vi "Draw Flat Top Textured Triangle.vi"(0 "Texture 3":T2, 4 "Texture 2":T2, 6 "Texture 1":T2, 8 "Point 3":T2, 9 "Point 2":T2, 10 "Point 1":T2, 11 "Pixel Data in":u32[][](array[numeric])) -> (3 "Pixel Data out":u32[][](array[numeric]))   [LabVIEW 2022 SP3]
uses:
  Point 2D.ctl
  Raster.lvlib
  Method.ctl
  <vilib>/picture/picture.llb/imagedata.ctl
panel:
  in  "Texture":T1
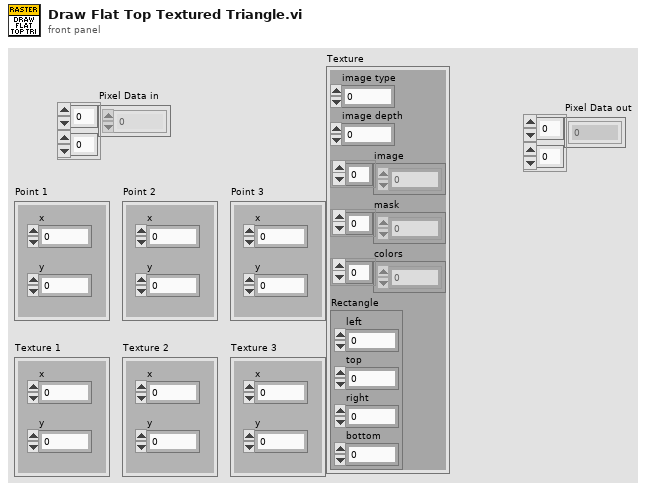
[diagram p1: front panel]
types:
  T1 = typedef "imagedata.ctl" = cluster{"image type":i32, "image depth":i32, "image":u8[], "mask":u8[], "colors":u32[], "Rectangle":cluster{"left":i16, "top":i16, "right":i16, "bottom":i16}}
  T2 = typedef "Raster.lvlib/Point 2D.ctl" = cluster{"x":i32, "y":i32}
  T3 = typedef "Raster.lvlib/Method.ctl" = enum16{"Per item", "Row", "Replace Array Subset", "MoveBlock", " MoveBlock2 "}
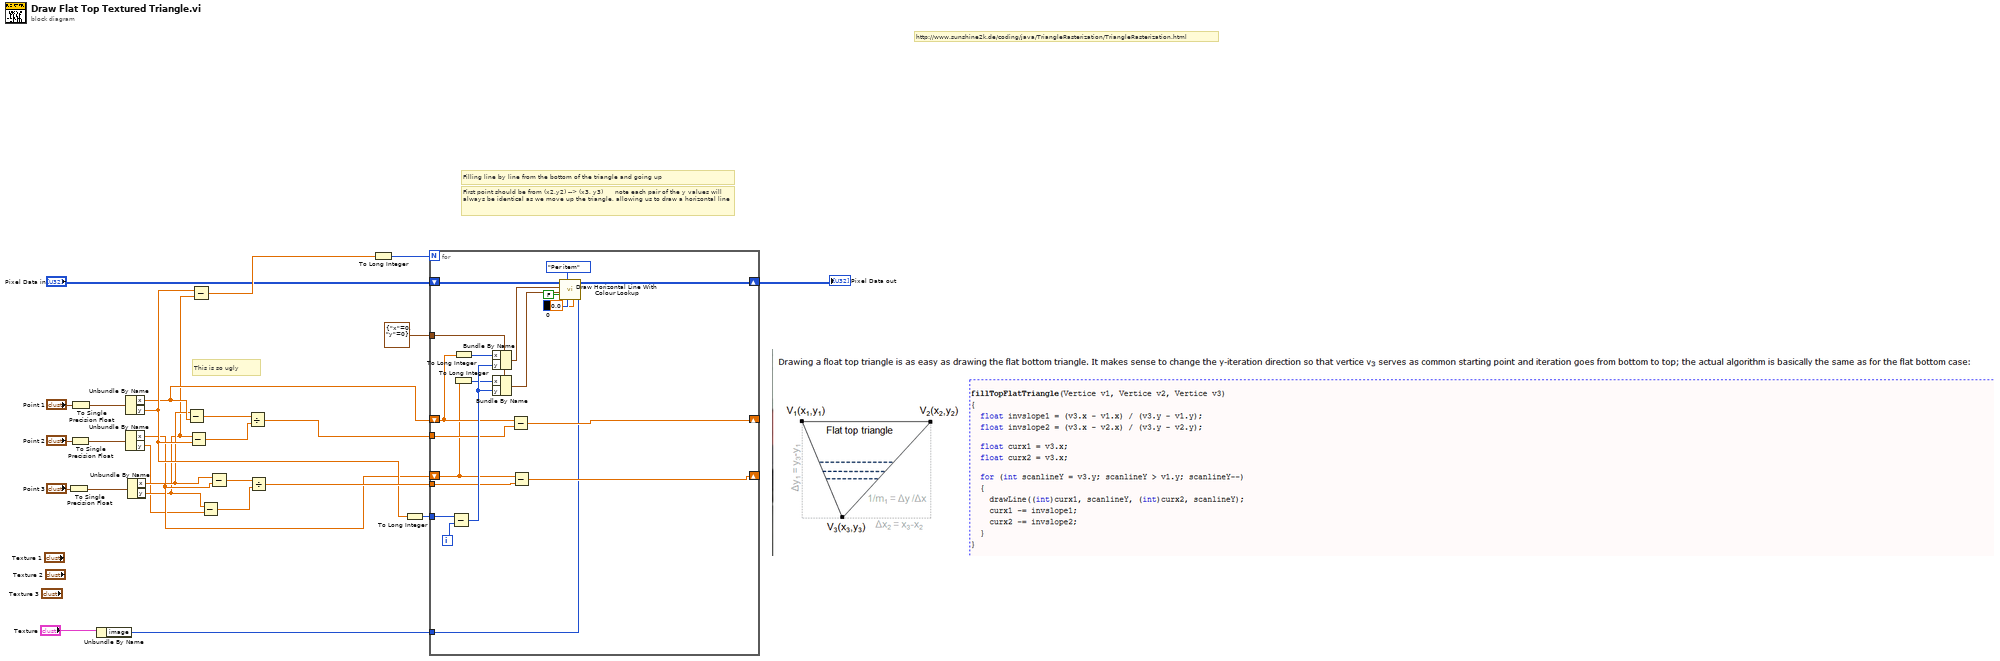
[diagram p0: block diagram]
diagram:
  # "This is so ugly"
  # "First point should be from (x2,y2) --> (x3, y3)      note each pair of the y values will always be identical as we move up the triangle, allowing us to draw a horizontal line"
  # "Filling line by line from the bottom of the triangle and going up"
  # "http://www.sunshine2k.de/coding/java/TriangleRasterization/TriangleRasterization.html"
  n1 = To Single Precision Float(number="Point 3") -> (single precision float=w19:cluster{"x":sgl, "y":sgl})
  n2 = To Single Precision Float(number="Point 2") -> (single precision float=w21:cluster{"x":sgl, "y":sgl})
  n3 = To Single Precision Float(number="Point 1") -> (single precision float=w23:cluster{"x":sgl, "y":sgl})
  n4 = Unbundle By Name("Texture") -> ("image"=w1:u8[])
  n5 = Unbundle By Name(w23) -> ("x"=w9:sgl, "y"=w10:sgl)
  n6 = Unbundle By Name(w21) -> ("x"=w7:sgl, "y"=w5:sgl)
  n7 = Unbundle By Name(w19) -> ("x"=w8:sgl, "y"=w6:sgl)
  n8 = Subtract(x=w8, y=w9) -> (x-y=w26:sgl)
  n9 = Subtract(x=w6, y=w10) -> (x-y=w17:sgl)
  n10 = Subtract(x=w10, y=w6) -> (x-y=w12:sgl)
  n11 = Subtract(x=w6, y=w5) -> (x-y=w18:sgl)
  n12 = Subtract(x=w8, y=w7) -> (x-y=w25:sgl)
  n13 = Divide(x=w26, y=w17) -> (x/y=w14:sgl)
  n14 = Divide(x=w25, y=w18) -> (x/y=w13:sgl)
  n15 = To Long Integer(number=w12) -> (32bit integer=w11:i32)
  n16 = To Long Integer(number=w10) -> (32bit integer=w15:i32)
  n17 = for {
    N: w11 -> [_]
    tunnel: T2 {"x"=0, "y"=0} ("Point 1") -> [w47]
    shift-right: [w37] -> _
    shift-left: w9 -> [w40]
    shift-right: [w38] -> _
    shift-left: w7 -> [w35]
    tunnel: w15 -> [w42]
    tunnel: w14 -> [w39]
    tunnel: w13 -> [w36]
    shift-right: [w32] -> w3
    shift-left: "Pixel Data in" -> [w33]
    tunnel: w1 -> [w27]
    i -> [w34]
    n18 = Subtract(x=w42, y=w34) -> (x-y=w43:i32)
    n19 = To Long Integer(number=w35) -> (32bit integer=w41:i32)
    n20 = To Long Integer(number=w40) -> (32bit integer=w44:i32)
    n21 = Bundle By Name(cluster=w47, "x"=w44, "y"=w43) -> (w46:T2)
    n22 = Bundle By Name(cluster=w47, "x"=w41, "y"=w43) -> (w45:T2)
    n23 = Subtract(x=w40, y=w39) -> (x-y=w37:sgl)
    n24 = Subtract(x=w35, y=w36) -> (x-y=w38:sgl)
    n25 = call "Draw Horizontal Line With Colour Lookup.vi"("Colours"=w27, "Alpha"=0.0, "Colour"=u32 0, "Method"=Method."Per item", "Enable Alpha Blending (F)"=FALSE, "Point 2"=w45, "Point 1"=w46, "Pixel Data in"=w33) -> ("Pixel Data out"=w32:u32[][])  [unwired: 3 in]
  }
  "Pixel Data out" <- w3
